vi "Get_recipe_Value_webserver.vi"() -> ()   [LabVIEW 2017]
uses:
  Generic_Common/Webserver/html_report_cluster.ctl
  <vilib>/httpClient/LabVIEWHTTPClient.lvlib
panel:
  out "StatusCodeName":string
  out "Session id name":string
  out "logout_url":string
  out "ErrorCode_expected":string
  out "Logout : Header  debug purpose":string
  out "Logout : Body debug purpose":string
  out "Status_message":string
  out "Logo":u16(ring)
  out "Iteration_Indicator":dbl
  out "Error code recieved":i32
  out "POST_command":string
  out "Command_url":string
  out "Test case":string
  out "Global ini path":path
  out "Test status":picture
  out "Time elapsed for each iteration":string
  out "DelayBetweenIterations":string
  out "Total_Iterations":i32
  out "Global_Webserver_Report":string
  out "TestSuite":string
  out "Error Out":errorcluster
  out "Response time":u32[](graph)
  out "Header of reponse for debug pupose":string
  out "Response from the web server":string
  # "AUTOMATION TESTING WEB SERVICES"
  # "TESTING DETAILS FROM INI"
  # "RESPONSE FROM WEBSERVER"
  # "ms"
  # "Webserver \n1. Webserver is being tested in this test case where SC board of ultrasonic welding machine is connected to test PC \t\t  \nSC IP address: 192.168.2.101, url=https://192.168.2.101\t\t\t\t\t\t\t\t\t\t \t\t\t  \n2. Ports used on SC board are as below:\t\t\t\t\t\t\t\t\t\t\t\t\t\t\t\t\t\t\t\t\t  \n   - J103: (Ethernet0) This port connected to UI controller large screen HMI display\trestricted webservices in this port\t\t\t\t\t\t\t\t\t  \n  - J104: (Ethernet1) This port is connected to local area network for accessing the webpage and testing  webserver                                \n  - J112: SC Logs are taken from this port. TeraTerm is configured  to this port so that SC logs are displayed on the screen."
  # "ms"
  # "RESPONSE TIME GRAPH"
  # "TESTING STATUS"
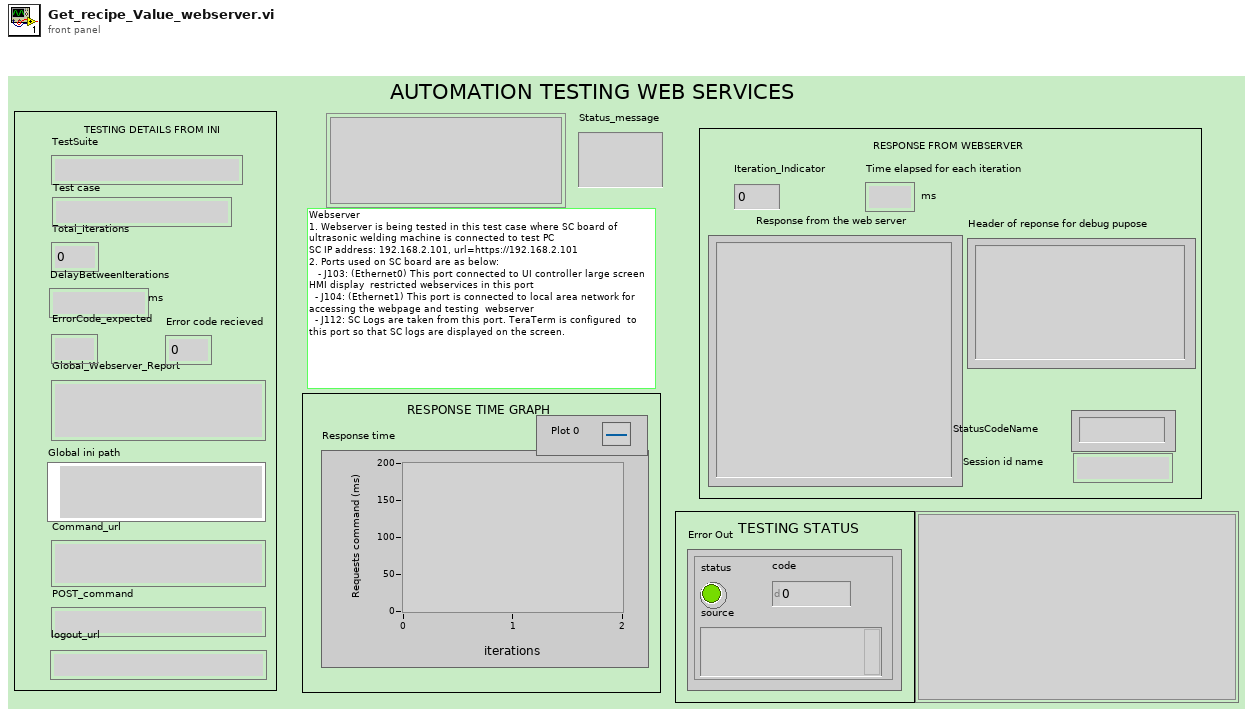
[diagram p1: front panel]
types:
  T1 = enum16{"open", "replace", "create", "open or create", "replace or create", "replace or create with confirmation"}
  T2 = enum8{"Enabled", "Disabled", "Disabled and Grayed Out"}
  T3 = cluster{"[0]":string, "[1]":string, "[2]":string, "[3]":string, "[4]":string, "[5]":string, "[6]":string, "[7]":string, "[8]":string}
  T4 = cluster{"login_url":string, "userid":string, "password":string, "command_url":string, "POST_command":string, "StatusCode_expected":string, "Iterations":string, "DelayBetweenIterations":string, "Timeout":string, "logout_url":string, "TestSuite":string}
  T5 = cluster{"Server_IP_Address":string, "Server_Port_Number":string, "Sid":string, "StatusCodeName":string, "Global_Webserver_Report":string}
  T6 = typedef "html_report_cluster.ctl" = cluster{"Remarks":string, "Verdict":string, "Status Code":i32, "Status Description":string, "JazzDashboardLink":string, "ReprtPath":string, "Timestamp":string, "TestSuite":string, "TestCase":string, "Iterations":i64, "Time taken to execute  test in msec":string, "Delay Between Iterations":i64}
  T7 = typedef "LabVIEWHTTPClient.lvlib/ClientHandle.ctl" = refnum<k1>
  T8 = typedef "imagedata.ctl" = cluster{"image type":i32, "image depth":i32, "image":u8[], "mask":u8[], "colors":u32[], "Rectangle":cluster{"left":i16, "top":i16, "right":i16, "bottom":i16}}
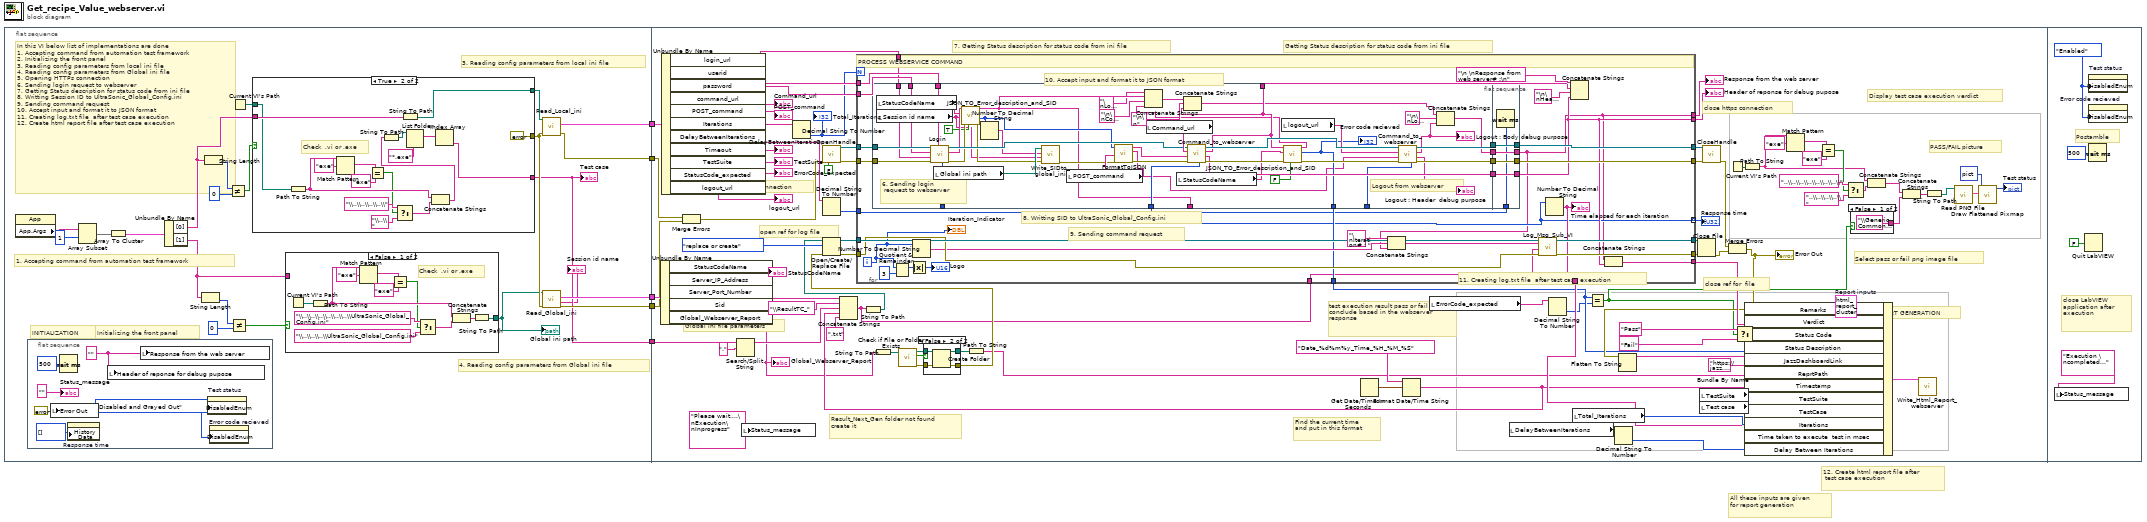
[diagram p0: block diagram]
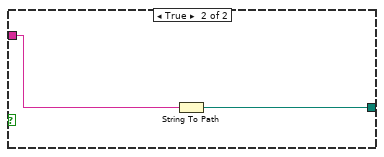
[diagram p2: hidden frame]
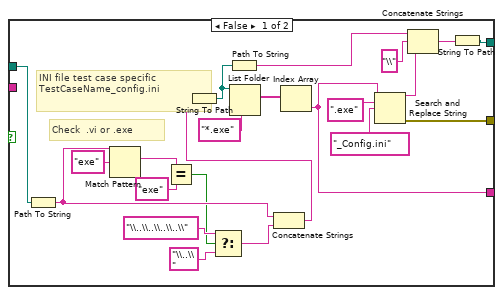
[diagram p3: hidden frame]
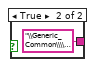
[diagram p5: hidden frame]
diagram:
  # "All these inputs are given \nfor report generation"
  # "12. Create html report file after\n test case execution"
  n1 = flat-sequence {
    tunnel: [w16] -> w5
    tunnel: [w19] -> w4
    tunnel: [w18] -> w3
    tunnel: [w17] -> w2
    tunnel: [w7] -> w1
    tunnel: w5 -> [w138]
    tunnel: w4 -> [w171]
    tunnel: w3 -> [w172]
    tunnel: w2 -> [w137]
    tunnel: w1 -> [w110]
    frame #0 {
      # "INITIALIZATION"
      # "4. Reading config parameters from Global ini file"
      # "3. Reading config parameters from local ini file"
      # "2. Initializing the front panel"
      # "1. Accepting command from automation test framework"
      # "In this VI below list of implementations are done\n1. Accepting command from automation test framework\n2. Initializing the front panel\n3. Reading config parameters from local ini file\n4. Reading config parameters from Global ini file\n5. Opening HTTPs connection\n6. Sending login request to webserver\n7. Getting Status description for status code from ini file\n8. Writting Session ID to UltraSonic_Global_Config.ini\n9. Sending command request\n10. Accept input and format it to JSON format\n11. Creating log.txt file  after test case execution\n12. Create html report file after test case execution"
      n2 = property class="App"() -> ("App.Args"=w21:string[])  [unwired: 2 in, 2 out]
      n3 = flat-sequence {
        frame #0 {
          w28 = T2."Disabled and Grayed Out" ("Disabled")
          w33 = ""
          n4 = local write "Error Out"(errorcluster {"status"=FALSE, "code"=0, "source"=""} ("error constant")) -> ()
          n5 = Wait (ms)(milliseconds to wait=u32 500) -> ()  [unwired: 1 out]
          n6 = property on="Response time" class="WFChart (strict)"("History Data"=u32[] []) -> ()  [unwired: 2 in, 2 out]
          n7 = local write "Header of reponse for debug pupose"(w33) -> ()
          n8 = local write "Response from the web server"(w33) -> ()
          n9 = property on="Test status" class="Pict"("DisabledEnum"=w28) -> ()  [unwired: 2 in, 2 out]
          n10 = property on="Error code recieved" class="DigNum (strict)"("DisabledEnum"=w28) -> ()  [unwired: 2 in, 2 out]
          "Status_message" <- ""
        }
      }
      n11 = Array Subset "Array Subset"(array=w21, index=1) -> (w22:string[])  [unwired: 1 in]
      n12 = Array To Cluster(array=w22) -> (cluster=w23:T3)
      n13 = Unbundle By Name "Unbundle By Name"(w23) -> ("[0]"=w15:string, "[1]"=w10:string)
      n14 = String Length(string=w10) -> (length=w27:i32)
      n15 = String Length(string=w15) -> (length=w24:i32)
      n16 = Not Equal?(x=w24, y=0) -> (x != y?=w13:bool)
      n17 = Not Equal?(x=w27, y=0) -> (x != y?=w11:bool)
      n18 = Current VI's Path() -> (path=w14:path)
      n19 = case shown="True" w13 {
        tunnel: w15 -> [_ w85]
        tunnel: [w61 w84] -> w8
        tunnel: [w60 errorcluster {"status"=FALSE, "code"=0, "source"=""} ("error out")] -> w12
        tunnel: w14 -> [w49 w70]
        tunnel: [w47 w69] -> w7
        frame False {
          # "Check  .vi or .exe"
          # "INI file test case specific\nTestCaseName_config.ini"
          n20 = Path To String(path=w49) -> (string=w54:string)
          n21 = Match Pattern(string=w54, regular expression="exe") -> (match substring=w53:string)  [unwired: 1 in, 3 out]
          n22 = Equal?(x=w53, y="exe") -> (x = y?=w51:bool)
          n23 = Select(t="\\..\\..\\..\\..\\" ("string"), s=w51, f="\\..\\" ("string")) -> (s? t:f=w55:string)
          n24 = Concatenate Strings(w54, w55) -> (w48:string)
          n25 = String To Path(string=w48) -> (path=w59:path)
          n26 = Path To String(path=w59) -> (string=w58:string)
          n27 = List Folder(path=w59, pattern="*.exe") -> (filenames=w62:string[])  [unwired: 2 in, 3 out]
          n28 = Index Array(array=w62) -> (element=w47:string)  [unwired: 1 in]
          n29 = Search and Replace String(input string=w47, search string=".exe", replace string="_Config.ini" ("replace string (\"\")")) -> (result string=w66:string, error out=w60:errorcluster)  [unwired: 5 in, 2 out]
          n30 = Concatenate Strings(w58, "\\" ("string"), w66) -> (w64:string)
          n31 = String To Path(string=w64) -> (path=w61:path)
        }
        frame True {
          # "Check  .vi or .exe"
          n32 = Path To String(path=w70) -> (string=w76:string)
          n33 = Match Pattern(string=w76, regular expression="exe") -> (match substring=w75:string)  [unwired: 1 in, 3 out]
          n34 = Equal?(x=w75, y="exe") -> (x = y?=w73:bool)
          n35 = Select(t="\\..\\..\\..\\..\\" ("string"), s=w73, f="\\..\\" ("string")) -> (s? t:f=w77:string)
          n36 = String To Path(string=w85) -> (path=w84:path)
          n37 = Concatenate Strings(w76, w77) -> (w71:string)
          n38 = String To Path(string=w71) -> (path=w80:path)
          n39 = List Folder(path=w80, pattern="*.exe") -> (filenames=w81:string[])  [unwired: 2 in, 3 out]
          n40 = Index Array(array=w81) -> (element=w69:string)  [unwired: 1 in]
        }
      }
      "Test case" <- w7
      n41 = case shown="False" w11 {
        tunnel: [w43 w46] -> w9
        tunnel: w10 -> [_ w45]
        frame False {
          # "Check  .vi or .exe"
          n42 = Current VI's Path() -> (path=w35:path)
          n43 = Path To String(path=w35) -> (string=w39:string)
          n44 = Match Pattern(string=w39, regular expression="exe") -> (match substring=w38:string)  [unwired: 1 in, 3 out]
          n45 = Equal?(x=w38, y="exe") -> (x = y?=w36:bool)
          n46 = Select(t="\\..\\..\\..\\..\\..\\..\\UltraSonic_Global_Config.ini" ("string"), s=w36, f="\\..\\..\\..\\UltraSonic_Global_Config.ini" ("string")) -> (s? t:f=w40:string)
          n47 = Concatenate Strings(w39, w40) -> (w44:string)
          n48 = String To Path(string=w44) -> (path=w43:path)
        }
        frame True {
          n49 = String To Path(string=w45) -> (path=w46:path)
        }
      }
      "Global ini path" <- w9
      n50 = call "Read_Local_ini.vi"("Error In"=w12, "Local ini path"=w8) -> ("Error Out"=w16:errorcluster, "Read from ini file"=w18:T4)  [unwired: 8 in]
      n51 = call "Read_Global_ini.vi"("Error In"=w12, "Global ini path"=w9) -> ("Error Out"=w17:errorcluster, "Session id name"=→"Session id name":string, "Global Cluster"=w19:T5)  [unwired: 7 in]
    }
    frame #1 {
      w154 = T6 {"Remarks"="", "Verdict"="", "Status Code"=0, "Status Description"="", "JazzDashboardLink"="", "ReprtPath"="", "Timestamp"="", "TestSuite"="", "TestCase"="", "Iterations"=0, "Time taken to execute  test in msec"="", "Delay Between Iterations"=1000}  # Report inputs
      # "Getting Status description for status code from ini file"
      # "7. Getting Status description for status code from ini file"
      # "Select pass or fail png image file"
      # "test execution result pass or fail\nconclude based in the webserver\nresponse"
      # "Find the current time \nand put in this format"
      # "open ref for log file"
      # "Result_Next_Gen folder not found\ncreate it"
      # "Global ini file parameters"
      # "local ini file parameters"
      # "close ref for  file"
      # "close https connection"
      # "Display test case execution verdict"
      # "11. Creating log.txt file  after test case execution"
      # "5. Opening HTTPs connection"
      # "REPORT GENERATION"
      # "PASS/FAIL picture"
      n52 = Unbundle By Name(w171) -> ("StatusCodeName"=→"StatusCodeName":string, "Global_Webserver_Report"=w102:string)  [unwired: 3 out]
      "Global_Webserver_Report" <- w102
      n53 = Unbundle By Name(w172) -> ("login_url"=w133:string, "userid"=w168:string, "password"=w167:string, "command_url"=→"Command_url":string, "POST_command"=→"POST_command":string, "Iterations"=w164:string, "DelayBetweenIterations"=w163:string, "TestSuite"=→"TestSuite":string, "StatusCode_expected"=→"ErrorCode_expected":string, "logout_url"=→"logout_url":string)  [unwired: 1 out]
      "DelayBetweenIterations" <- w163
      n54 = Merge Errors(w138, w137) -> (w136:errorcluster)
      n55 = Search/Split String(string=w110, search string/char (-)=".") -> (substring before match=w108:string)  [unwired: 1 in, 2 out]
      n56 = local write "Status_message"("Please wait....\nExecution\nInprogress") -> ()
      n57 = Decimal String To Number(string=w164) -> (number=w152:i32)  [unwired: 2 in, 1 out]
      "Total_Iterations" <- w152
      n58 = call <vilib>:"OpenHandle.vi"("error in (no error)"=w136, "verify server(true)"=FALSE) -> ("client handle out"=w170:T7, "error out"=w169:errorcluster)  [unwired: 12 in]
      n59 = Decimal String To Number(string=w163) -> (number=w162:i32)  [unwired: 2 in, 1 out]
      n60 = String To Path(string=w102) -> (path=w107:path)
      n61 = call <vilib>:"Check if File or Folder Exists.vi"("path"=w107) -> ("error out"=w103:errorcluster, "file or folder exists?"=w106:bool, "dup path"=w105:path)  [unwired: 8 in]
      n62 = case shown="False" w106 {
        tunnel: [w173 w178] -> w101
        tunnel: w105 -> [w174 w177]
        tunnel: [w174 w176] -> w104
        tunnel: w103 -> [w173 w175]
        frame True {
        }
        frame False {
          n63 = Create Folder(path (use dialog)=w177, error in=w175) -> (created path=w176:path, error out=w178:errorcluster)  [unwired: 1 in, 1 out]
        }
      }
      n64 = Path To String(path=w104) -> (string=w100:string)
      n65 = Get Date/Time In Seconds() -> (seconds since 1Jan1904=w88:timestamp)
      n66 = Format Date/Time String(time format string (%c)="Date_%d%m%y_Time_%H_%M_%S", seconds (now)=w88) -> (date/time string=w113:string)  [unwired: 1 in]
      n67 = Concatenate Strings(w102, "\\ResultTC_" ("string"), w108, w113, ".txt" ("string")) -> (w87:string)
      n68 = String To Path(string=w87) -> (path=w111:path)
      n69 = Open/Create/Replace File(file path (use dialog)=w111, error in=w101, operation (0:open)=T1."replace or create") -> (refnum out=w161:refnum<file>, error out=w160:errorcluster)  [unwired: 3 in, 1 out]
      n70 = for {
        N: w152 -> [_]
        tunnel: w170 -> [w213]
        tunnel: w167 -> [w210]
        tunnel: [w181] -> w166
        tunnel: w168 -> [w211]
        tunnel: [w195] -> w165
        tunnel: w169 -> [w212]
        tunnel: w162 -> [w188]
        tunnel: [w182] -> w145 mode=indexing
        tunnel: w161 -> [w208]
        tunnel: w160 -> [w207]
        tunnel: [w206] -> w159
        tunnel: [w205] -> w158
        tunnel: [w201] -> w156
        tunnel: [w200] -> w155
        tunnel: [w196] -> w143
        tunnel: w133 -> [w198]
        tunnel: [w194] -> w115
        tunnel: [w189] -> w93
        tunnel: w87 -> [w183]
        i -> [w191]
        # "8. Writting SID to UltraSonic_Global_Config.ini"
        # "10. Accept input and format it to JSON format"
        # "9. Sending command request"
        # "PROCESS WEBSERVICE COMMAND"
        n71 = flat-sequence {
          tunnel: w211 -> [w257]
          tunnel: w210 -> [w256]
          tunnel: [w214] -> w187
          tunnel: [w244] -> w186
          tunnel: [w247] -> w185
          tunnel: [w245] -> w184
          tunnel: w198 -> [w255]
          tunnel: [w231] -> w197
          tunnel: [w228] -> w189
          tunnel: [w230] -> _
          tunnel: [w235] -> _
          tunnel: [w234] -> w182
          tunnel: [w233] -> _
          tunnel: w213 -> [w259]
          tunnel: w212 -> [w258]
          tunnel: [w261] -> w200
          tunnel: [w262] -> w201
          tunnel: [w263] -> w195
          tunnel: [w264] -> w181
          tunnel: w187 -> [w264]
          tunnel: w186 -> [w263]
          tunnel: w185 -> [w262]
          tunnel: w184 -> [w261]
          tunnel: w188 -> [w260]
          frame #0 {
            # "Logout from webserver"
            # "6. Sending login\n request to webserver"
            n72 = local read "StatusCodeName"() -> (w223:string)
            n73 = local read "Session id name"() -> (w222:string)
            n74 = call "Login.vi"("userid"=w257, "Error In"=w258, "Command to webservice"=w255, "password"=w256, "IN HTTPS client handle"=w259) -> ("Error Out"=w238:errorcluster, "Body of reponse"=w229:string, "OUT HTTPS client handle"=w251:T7, "Response time"=w233:u32)  [unwired: 2 in, 1 out]
            n75 = local read "Global ini path"() -> (w242:path)
            n76 = call "JSON_TO_Error_description_and_SID.vi"("Sid_present_in_webserver_response"=TRUE, "Error In"=w238, "Session id name"=w222, "Status code name"=w223, "JSON String input"=w229) -> ("Error Out"=w237:errorcluster, "SID"=w240:i32, "status_selected"=w230:string)  [unwired: 3 in, 1 out]
            n77 = Number To Decimal String(number=w240) -> (decimal integer string=w239:string)  [unwired: 1 in]
            n78 = call "Write_SIDto_global_ini.vi"("Error In"=w237, "Session id name"=w222, "SID"=w239, "Global ini path"=w242) -> ("Error Out"=w241:errorcluster)  [unwired: 7 in]
            n79 = local read "POST_command"() -> (w254:string)
            n80 = call "FormatToJSON.vi"("Error In"=w241, "Post_command"=w254, "Sid"=w240) -> ("Error Out"=w253:errorcluster, "POST_command_sid_only"=w218:string, "Final_POST_Command"=w219:string)  [unwired: 6 in]
            n81 = local read "Command_url"() -> (w252:string)
            n82 = local read "StatusCodeName"() -> (w220:string)
            n83 = call "Command_to_webserver.vi"("Error In"=w253, "JSON post command"=w219, "URL Command to Logout"=w252, "https client handle in ref"=w251) -> ("Error Out"=w249:errorcluster, "Header of response for debug purpose"=w244:string, "Body of response"=w231:string, "https client handle out ref"=w246:T7, "Reponse time"=w234:u32)  [unwired: 3 in]
            n84 = local read "logout_url"() -> (w236:string)
            n85 = call "JSON_TO_Error_description_and_SID.vi"("Sid_present_in_webserver_response"=FALSE, "Error In"=w249, "Status code name"=w220, "JSON String input"=w231) -> ("Error Out"=w248:errorcluster, "status code"=w228:i32, "status_selected"=w226:string)  [unwired: 4 in, 1 out]
            "Error code recieved" <- w228
            n86 = Concatenate Strings("\nLogin:\n" ("string"), w230, "\n\nCommand : Status Code description\n" ("string"), w226) -> (w232:string)
            n87 = Concatenate Strings(w232, "\n\n", w231) -> (w215:string)
            n88 = call "Command_to_webserver.vi"("Error In"=w248, "JSON post command"=w218, "URL Command to Logout"=w236, "https client handle in ref"=w246) -> ("Error Out"=w247:errorcluster, "Header of response for debug purpose"=→"Logout : Header  debug purpose":string, "Body of response"=w216:string, "https client handle out ref"=w245:T7, "Reponse time"=w235:u32)  [unwired: 3 in]
            "Logout : Body debug purpose" <- w216
            n89 = Concatenate Strings(w215, "\n\nLogout:\n" ("string"), w216) -> (w214:string)
          }
          frame #1 {
            n90 = Wait (ms)(milliseconds to wait=w260) -> ()  [unwired: 1 out]
          }
        }
        n91 = Quotient & Remainder(x=w191, y=3) -> (x-y*floor(x/y)=w192:i32)  [unwired: 1 out]
        n92 = Absolute Value(x=w192) -> (abs(x)=→"Logo":i32)
        n93 = Number To Decimal String(number=w191) -> (decimal integer string=w202:string)  [unwired: 1 in]
        n94 = Concatenate Strings("\nIteration# : " ("string"), w202, w181) -> (w204:string)
        n95 = call "Log_Msg_Sub_VI.vi"("Error In"=w207, "Path for CSV"=w183, "String input"=w204, "refnum in"=w208) -> ("Error Out"=w205:errorcluster, "refnum out"=w206:refnum<file>)  [unwired: 6 in]
        n96 = Number To Decimal String(number=w182) -> (decimal integer string=w194:string)  [unwired: 1 in]
        "Time elapsed for each iteration" <- w194
        n97 = Concatenate Strings("\n \nResponse from web server# :\n" ("string"), w197, "\n\nHeader# : \n", w195) -> ()  [unwired: 1 out]
        n98 = Concatenate Strings(w181, w195) -> (w196:string)
        "Iteration_Indicator" <- w191
      }
      "Response from the web server" <- w166
      "Header of reponse for debug pupose" <- w165
      "Response time" <- w145
      n99 = local read "ErrorCode_expected"() -> (w94:string)
      n100 = local read "DelayBetweenIterations"() -> (w147:string)
      n101 = Decimal String To Number(string=w94) -> (number=w92:i32)  [unwired: 2 in, 1 out]
      n102 = local read "Total_Iterations"() -> (w148:i32)
      n103 = Equal?(x=w93, y=w92) -> (x = y?=w91:bool)
      n104 = Decimal String To Number(string=w147) -> (number=w146:i32)  [unwired: 2 in, 1 out]
      n105 = Close File(refnum=w159, error in=w158) -> (error out=w150:errorcluster)  [unwired: 1 out]
      n106 = local read "TestSuite"() -> (w149:string)
      n107 = local read "Test case"() -> (w135:string)
      n108 = call <vilib>:"CloseHandle.vi"("client handle"=w155, "error in (no error)"=w156) -> ("error out"=w151:errorcluster)  [unwired: 13 in]
      n109 = Current VI's Path() -> (path=w121:path)
      n110 = Merge Errors(w151, w150) -> (w99:errorcluster)
      "Error Out" <- w99
      n111 = Flatten To String(anything=w99) -> (data string=w98:string)  [unwired: 3 in, 2 out]
      n112 = Select(t="Pass", s=w91, f="Fail") -> (s? t:f=w140:string)
      n113 = Path To String(path=w121) -> (string=w119:string)
      n114 = Bundle By Name(cluster=w154, "Remarks"=w143, "Verdict"=w140, "Status Code"=w93, "Status Description"=w98, "JazzDashboardLink"="https://jazz.bucclm.com/", "ReprtPath"=w100, "Timestamp"=w113, "TestSuite"=w149, "TestCase"=w135, "Iterations"=w148, "Time taken to execute  test in msec"=w115, "Delay Between Iterations"=w146) -> (w153:T6)
      n115 = Match Pattern(string=w119, regular expression="exe") -> (match substring=w125:string)  [unwired: 1 in, 3 out]
      n116 = Equal?(x=w125, y="exe") -> (x = y?=w123:bool)
      n117 = Select(t="..\\..\\..\\..\\..\\..\\..\\" ("string"), s=w123, f="..\\..\\..\\..\\" ("string")) -> (s? t:f=w120:string)
      n118 = case shown="False" w91 {
        tunnel: ["\\Generic_Common\\\\Webserver\\\\Fail.png" "\\Generic_Common\\\\Webserver\\\\Pass.png"] -> w129
        frame False {
        }
        frame True {
        }
      }
      n119 = Concatenate Strings(w119, w120) -> (w118:string)
      n120 = Concatenate Strings(w118, w129) -> (w128:string)
      n121 = call "Write_Html_Report_webserver.vi"("Report inputs"=w153) -> ()  [unwired: 18 in, 1 out]
      n122 = String To Path(string=w128) -> (path=w117:path)
      n123 = call <vilib>:"Read PNG File.vi"("path to PNG file"=w117) -> ("image data"=w116:T8)  [unwired: 8 in, 2 out]
      n124 = call <vilib>:"Draw Flattened Pixmap.vi"("image data"=w116, "picture"=picture data[5B]) -> ("new picture"=→"Test status":picture)  [unwired: 7 in]
    }
    frame #2 {
      w265 = T2."Enabled" ("Disabled")
      # "close LabVIEW \napplication after \nexecution"
      # "Postamble"
      n125 = local write "Status_message"("Execution \ncompleted...") -> ()
      n126 = Quit LabVIEW(quit? (T)=FALSE) -> ()
      n127 = property on="Test status" class="Pict"("DisabledEnum"=w265) -> ()  [unwired: 2 in, 2 out]
      n128 = property on="Error code recieved" class="DigNum (strict)"("DisabledEnum"=w265) -> ()  [unwired: 2 in, 2 out]
      n129 = Wait (ms)(milliseconds to wait=u32 500) -> ()  [unwired: 1 out]
    }
  }
